vi "335 Read and Compressor auto control(SubVI).vi"(6 "压缩机自动停机":bool, 9 "自动控制":bool, 10 "数值":i32, 11 "Instrument":T1={"335 Resource"="", "Input (0:A)"=0, "Instrument Type"=enum."PPMS", "quantum design"=refnum, "Heater Output (1:1)"=0, "semaphore"=refnum, "TCP master instance"=refnum, "335 Status"=refnum, "M24C Resource"="GPIB0::24::INSTR", "4G supply"="GPIB0::24::INSTR", "Temp Status 24C"=refnum, "4g supply status"=refnum, "Temp"=refnum} {"Input (0:A)" items=["A", "B"]; "Heater Output (1:1)" items=["1"=1, "2"=2]}) -> (3 "簇":T5 {"?" items=["Unknow", "Stable", "Following Warm", "Following Cold", "Unfollowing"]})   [LabVIEW 2019, in "Get value.lvlib"]
uses:
  Get value.lvlib
  335 state.ctl
  Instrument.ctl
  <vilib>/NI/Modbus Library/API/Master/Modbus Master.lvclass
  Instrument Type.ctl
  lib/QDInstrument.dll
  lib/Lake Shore 335/Lake Shore 335.lvlib
panel:
  out "error out":errorcluster
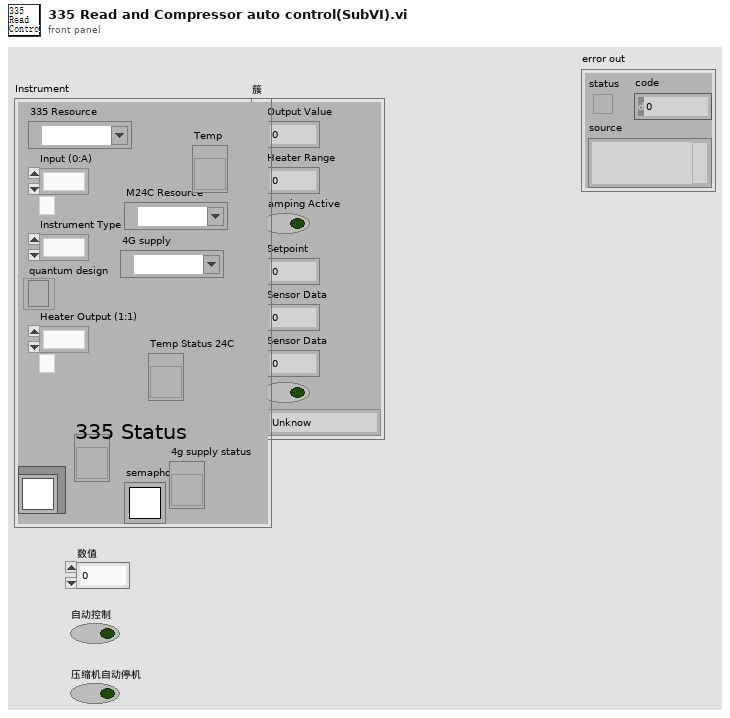
[diagram p1: front panel]
types:
  T1 = typedef "Instrument.ctl" = cluster{"335 Resource":refnum<visa-resource-name>, "Input (0:A)":u16, "Instrument Type":T2, "quantum design":refnum<k24>, "Heater Output (1:1)":u16, "semaphore":T3, "TCP master instance":refnum<class "Modbus Master.lvclass">, "335 Status":refnum<vi>, "M24C Resource":refnum<visa-resource-name>, "4G supply":refnum<visa-resource-name>, "Temp Status 24C":refnum<vi>, "4g supply status":refnum<vi>, "Temp":refnum<vi>}
  T2 = typedef "Instrument Type.ctl" = enum16{"PPMS", "VersaLab", "DynaCool", "SVSM", "PPMS-Rotate", "Lakeshore335", "9T mag"}
  T3 = typedef "Semaphore RefNum" = refnum<k1>
  T4 = typedef "335 state.ctl" = u16
  T5 = cluster{"Output Value":dbl, "Heater Range ":u16, "Ramping Active":bool, "Setpoint":dbl, "Sensor Data":dbl, "Sensor Data":dbl, bool, T4}
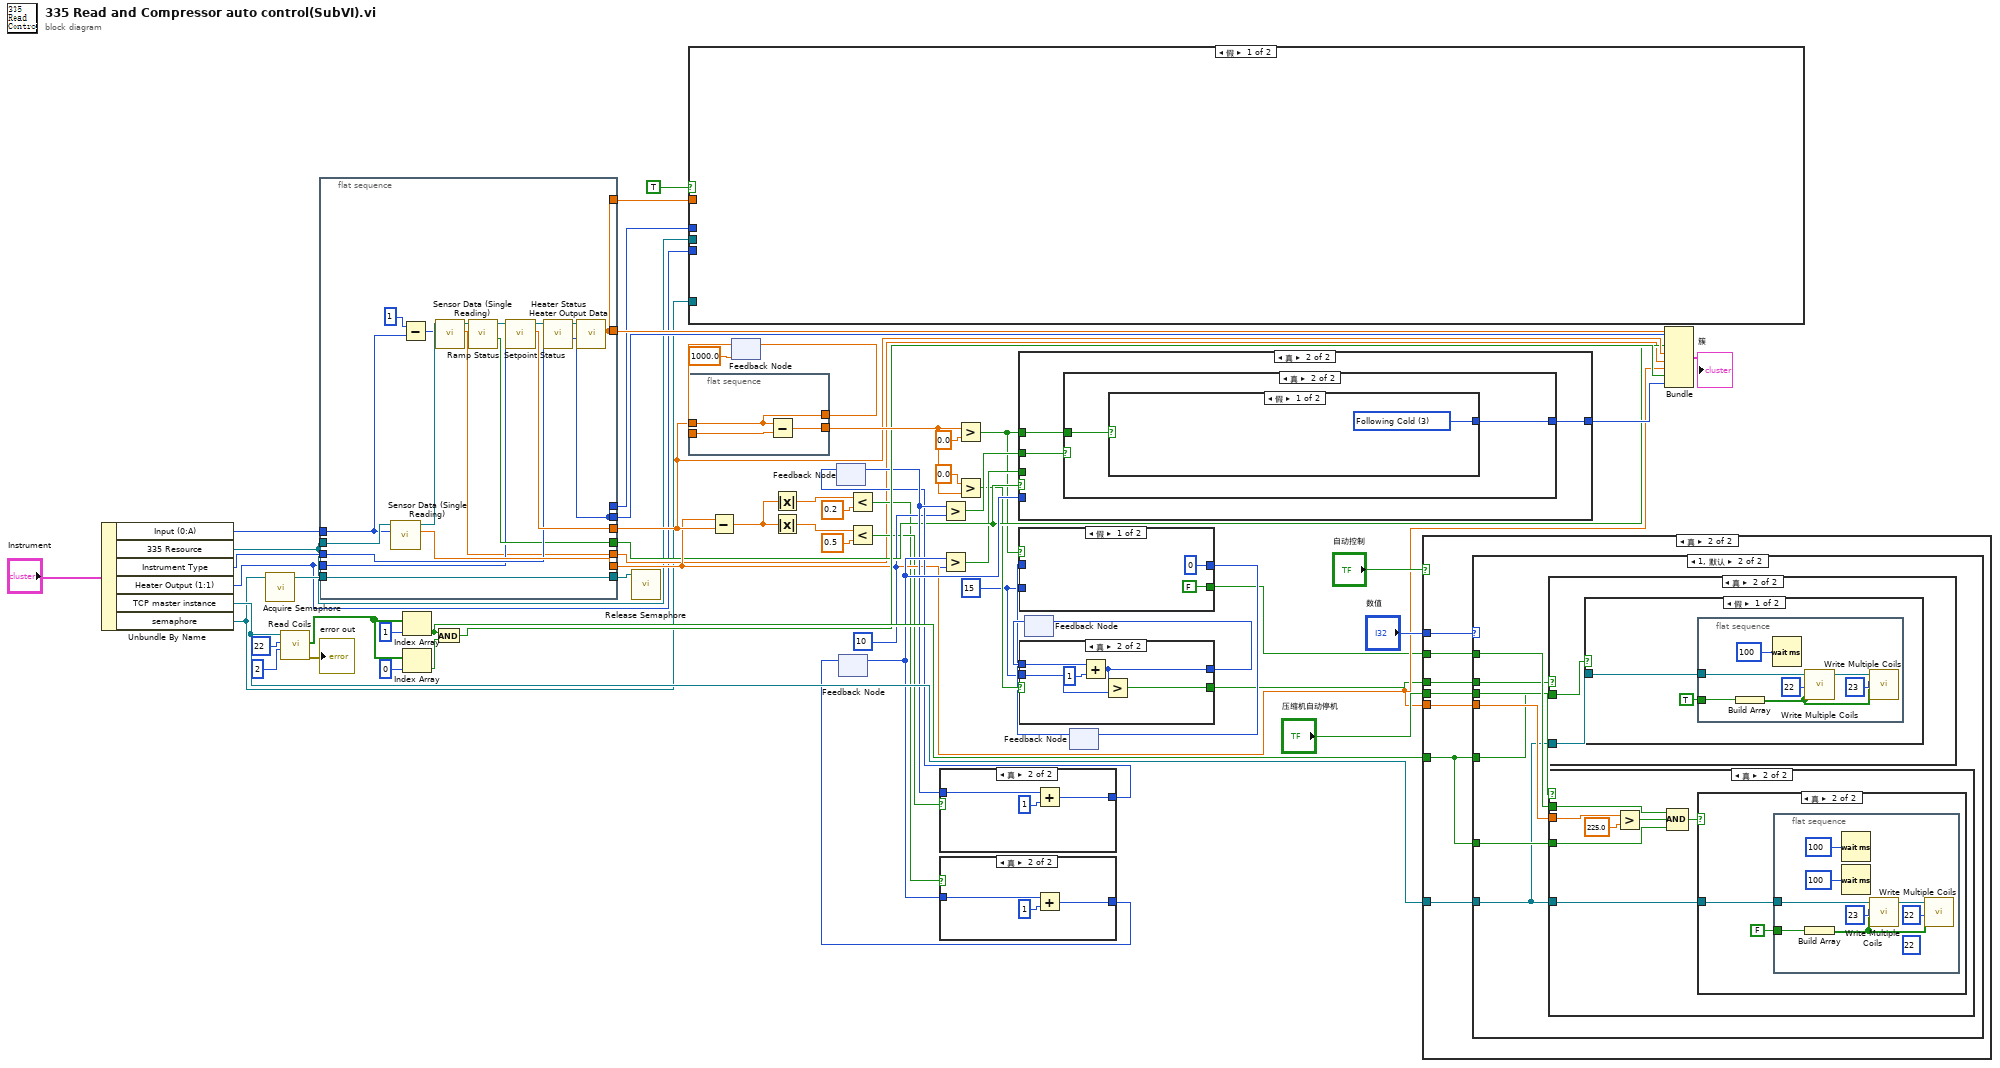
[diagram p0: block diagram]
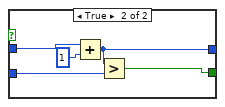
[diagram p2: hidden frame]
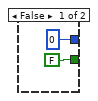
[diagram p3: hidden frame]
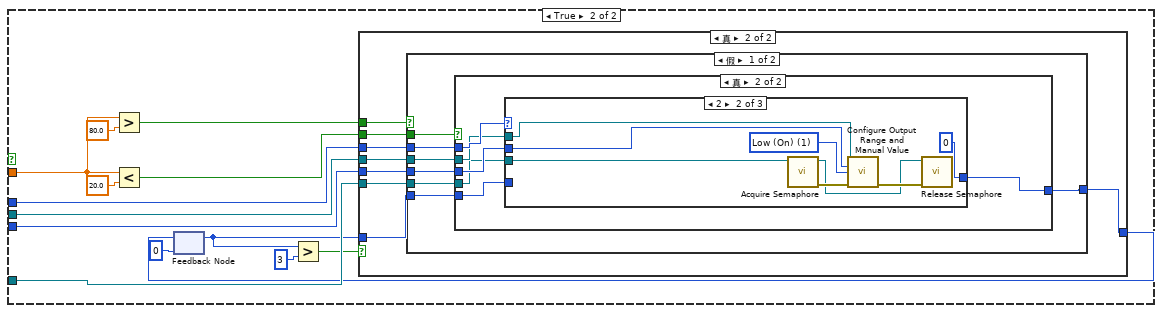
[diagram p4: hidden frame]
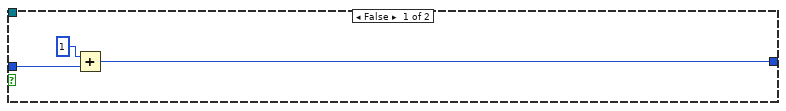
[diagram p5: hidden frame]
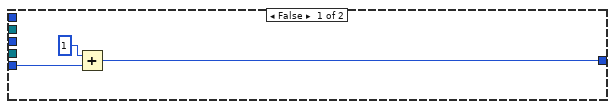
[diagram p6: hidden frame]
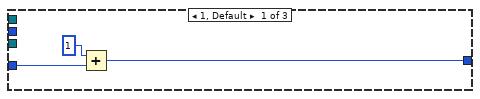
[diagram p7: hidden frame]
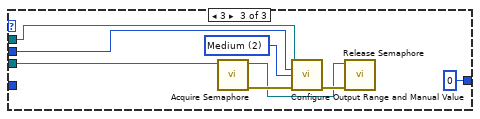
[diagram p8: hidden frame]
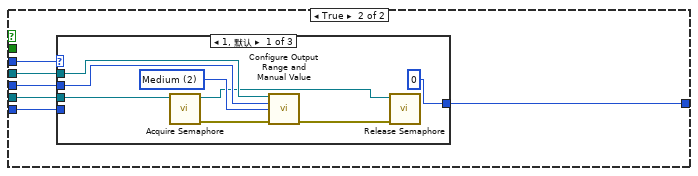
[diagram p9: hidden frame]
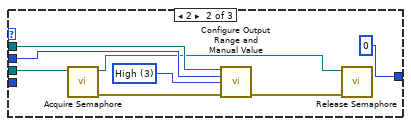
[diagram p10: hidden frame]
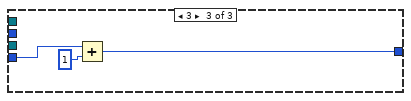
[diagram p11: hidden frame]
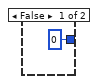
[diagram p18: hidden frame]
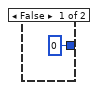
[diagram p19: hidden frame]
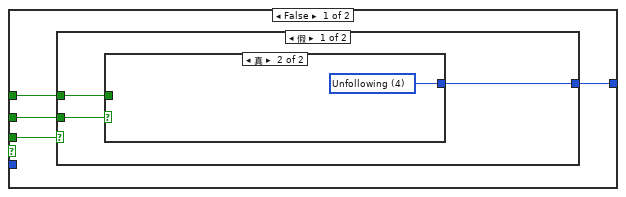
[diagram p20: hidden frame]
diagram:
  w2 = 15 ("y")
  w35 = 10 ("y")
  n1 = Unbundle By Name("Instrument") -> ("Input (0:A)"=w21:u16, "335 Resource"=w13:refnum<visa-resource-name>, "Instrument Type"=w18:T2, "Heater Output (1:1)"=w12:u16, "TCP master instance"=w59:refnum<class "Modbus Master.lvclass">, "semaphore"=w11:T3)
  n2 = call <vilib>:"Acquire Semaphore.vi"("semaphore"=w11) -> ("semaphore out"=w19:T3)  [unwired: 4 in, 2 out]
  n3 = call-dynamic "Read Coils.vi"("number of inputs"=u16 2, "starting address"=u16 22, "Modbus master in"=w59) -> ("error out"=→"error out":errorcluster, "coils"=w48:bool[])  [unwired: 6 in, 1 out]
  n4 = flat-sequence {
    tunnel: [w79] -> w49
    tunnel: w13 -> [w77]
    tunnel: [w74] -> w39
    tunnel: w18 -> [w73]
    tunnel: w19 -> [w72]
    tunnel: [w72] -> w20
    tunnel: [w62] -> w23
    tunnel: [w63] -> w22
    tunnel: [w71] -> w38
    tunnel: w12 -> [w70]
    tunnel: w21 -> [w69]
    tunnel: [w64] -> w24
    tunnel: [w63] -> w15
    tunnel: [w62] -> w14
    frame #0 {
      n5 = call "Sensor Data (Single Reading).vi"("Input (0:A)"=w69, "VISA resource name"=w77) -> ("Sensor Data"=w74:dbl, "VISA resource name out"=w67:refnum<visa-resource-name>)  [unwired: 7 in, 1 out]
      n6 = Subtract(x=u16 1, y=w69) -> (x-y=w65:u16)
      n7 = call "Sensor Data (Single Reading).vi"("Input (0:A)"=w65, "VISA resource name"=w67) -> ("Sensor Data"=w64:dbl, "VISA resource name out"=w66:refnum<visa-resource-name>)  [unwired: 7 in, 1 out]
      n8 = call "Ramp Status.vi"("VISA resource name"=w66) -> ("Ramping Active"=w71:bool, "VISA resource name out"=w78:refnum<visa-resource-name>)  [unwired: 6 in, 3 out]
      n9 = call "Setpoint Status.vi"("Output (1:1)"=w70, "VISA resource name"=w78) -> ("Setpoint"=w79:dbl, "VISA resource name out"=w76:refnum<visa-resource-name>)  [unwired: 7 in, 1 out]
      n10 = call "Heater Status.vi"("Heater Output (1:1)"=w73, "VISA resource name"=w76) -> ("Heater Range"=w62:u16, "VISA resource name out"=w75:refnum<visa-resource-name>)  [unwired: 5 in, 3 out]
      n11 = call "Heater Output Data.vi"("VISA resource name"=w75) -> ("Output Value"=w63:dbl)  [unwired: 8 in, 2 out]
    }
  }
  n12 = Index Array(array=w48, index=1) -> (element=w58:bool)
  n13 = Index Array(array=w48, index=0) -> (element=w44:bool)
  n14 = And(x=w58, y=w44) -> (x .and. y?=w45:bool)
  n15 = call <vilib>:"Release Semaphore.vi"("semaphore"=w20) -> ()  [unwired: 5 in, 2 out]
  n16 = case shown="假" TRUE {
    tunnel: w15 -> [_ w92]
    tunnel: w14 -> [_ w89]
    tunnel: w13 -> [_ w88]
    tunnel: w12 -> [_ w87]
    tunnel: w11 -> [_ w86]
    frame False {
    }
    frame True {
      n17 = Greater?(x=w92, y=80.0) -> (0:w90:bool)
      n18 = Less?(x=w92, y=20.0) -> (x < y?=w81:bool)
      n19 = feedback #1(0) -> (w82:i32)
      n20 = Greater?(x=w82, y=3) -> (0:w84:bool)
      n21 = case shown="真" w84 {
        tunnel: w90 -> [_ w104]
        tunnel: w89 -> [_ w103]
        tunnel: w88 -> [_ w102]
        tunnel: w87 -> [_ w101]
        tunnel: w86 -> [_ w100]
        tunnel: [w94 w99] -> w83
        tunnel: w82 -> [w96 w98]
        tunnel: w81 -> [_ w97]
        frame False {
          n22 = Add(x=1, y=w96) -> (x+y=w94:i32)
        }
        frame True {
          n23 = case shown="假" w104 {
            tunnel: w103 -> [w111 w145]
            tunnel: w102 -> [w110 w144]
            tunnel: w101 -> [w109 w143]
            tunnel: w100 -> [w106 w142]
            tunnel: [w108 w141] -> w99
            tunnel: w98 -> [w107 w140]
            tunnel: w97 -> [w105 _]
            frame False {
              n24 = case shown="真" w105 {
                tunnel: w111 -> [_ w120]
                tunnel: w110 -> [_ w119]
                tunnel: w109 -> [_ w118]
                tunnel: [w112 w117] -> w108
                tunnel: w107 -> [w114 w116]
                tunnel: w106 -> [_ w115]
                frame False {
                  n25 = Add(x=1, y=w114) -> (x+y=w112:i32)
                }
                frame True {
                  n26 = case shown="2" w120 {
                    tunnel: w119 -> [_ w127 w135]
                    tunnel: w118 -> [_ w126 w134]
                    tunnel: [w121 0 0] -> w117
                    tunnel: w116 -> [w123 _ _]
                    tunnel: w115 -> [_ w124 w132]
                    frame 1, Default {
                      n27 = Add(x=1, y=w123) -> (x+y=w121:i32)
                    }
                    frame 2 {
                      w131 = u16 1 items=["Off", "Low (On)", "Medium", "High"] ("Range (0:Off)")
                      n28 = call <vilib>:"Acquire Semaphore.vi"("semaphore"=w124) -> ("error out"=w130:errorcluster, "semaphore out"=w128:T3)  [unwired: 4 in, 1 out]
                      n29 = call "Configure Output Range and Manual Value.vi"("VISA resource name"=w127, "Heater Output (1:1)"=w126, "Range (0:Off)"=w131, "error in (no error)"=w130) -> ("error out"=w129:errorcluster)  [unwired: 10 in, 1 out]
                      n30 = call <vilib>:"Release Semaphore.vi"("error in (no error)"=w129, "semaphore"=w128) -> ()  [unwired: 4 in, 2 out]
                    }
                    frame 3 {
                      w139 = u16 2 items=["Off", "Low (On)", "Medium", "High"] ("Range (0:Off)")
                      n31 = call <vilib>:"Acquire Semaphore.vi"("semaphore"=w132) -> ("error out"=w138:errorcluster, "semaphore out"=w136:T3)  [unwired: 4 in, 1 out]
                      n32 = call "Configure Output Range and Manual Value.vi"("VISA resource name"=w135, "Heater Output (1:1)"=w134, "Range (0:Off)"=w139, "error in (no error)"=w138) -> ("error out"=w137:errorcluster)  [unwired: 10 in, 1 out]
                      n33 = call <vilib>:"Release Semaphore.vi"("error in (no error)"=w137, "semaphore"=w136) -> ()  [unwired: 4 in, 2 out]
                    }
                  }
                }
              }
            }
            frame True {
              n34 = case shown="1, 默认" w145 {
                tunnel: w144 -> [w153 w161 _]
                tunnel: w143 -> [w152 w160 _]
                tunnel: w142 -> [w146 w155 _]
                tunnel: [0 0 w162] -> w141
                tunnel: w140 -> [_ _ w164]
                frame 1, Default {
                  w149 = u16 2 items=["Off", "Low (On)", "Medium", "High"] ("Range (0:Off)")
                  n35 = call <vilib>:"Acquire Semaphore.vi"("semaphore"=w146) -> ("error out"=w150:errorcluster, "semaphore out"=w148:T3)  [unwired: 4 in, 1 out]
                  n36 = call "Configure Output Range and Manual Value.vi"("VISA resource name"=w153, "Heater Output (1:1)"=w152, "Range (0:Off)"=w149, "error in (no error)"=w150) -> ("error out"=w151:errorcluster)  [unwired: 10 in, 1 out]
                  n37 = call <vilib>:"Release Semaphore.vi"("error in (no error)"=w151, "semaphore"=w148) -> ()  [unwired: 4 in, 2 out]
                }
                frame 2 {
                  w159 = u16 3 items=["Off", "Low (On)", "Medium", "High"] ("Range (0:Off)")
                  n38 = call <vilib>:"Acquire Semaphore.vi"("semaphore"=w155) -> ("error out"=w158:errorcluster, "semaphore out"=w156:T3)  [unwired: 4 in, 1 out]
                  n39 = call "Configure Output Range and Manual Value.vi"("VISA resource name"=w161, "Heater Output (1:1)"=w160, "Range (0:Off)"=w159, "error in (no error)"=w158) -> ("error out"=w157:errorcluster)  [unwired: 10 in, 1 out]
                  n40 = call <vilib>:"Release Semaphore.vi"("error in (no error)"=w157, "semaphore"=w156) -> ()  [unwired: 4 in, 2 out]
                }
                frame 3 {
                  n41 = Add(x=w164, y=1) -> (x+y=w162:i32)
                }
              }
            }
          }
        }
      }
      n42 = feedback-in #1(w83) -> ()
    }
  }
  n43 = flat-sequence {
    tunnel: w49 -> [w167]
    tunnel: [w167] -> w50
    tunnel: w51 -> [w166]
    tunnel: [w165] -> w57
    frame #0 {
      n44 = Subtract(x=w167, y=w166) -> (x-y=w165:dbl)
    }
  }
  n45 = Subtract(x=w39, y=w49) -> (x-y=w33:dbl)
  n46 = feedback #2(1000.0 ("Setpoint")) -> (w51:dbl)
  n47 = feedback-in #2(w50) -> ()
  n48 = Absolute Value(x=w33) -> (abs(x)=w30:dbl)
  n49 = Absolute Value(x=w33) -> (abs(x)=w31:dbl)
  n50 = feedback #3() -> (w41:i32)  [unwired: 1 in]
  n51 = feedback #4() -> (w43:i32)  [unwired: 1 in]
  n52 = Less?(x=w30, y=0.2) -> (x < y?=w29:bool)
  n53 = Less?(x=w31, y=0.5) -> (x < y?=w34:bool)
  n54 = case shown="真" w34 {
    tunnel: w41 -> [_ w171]
    tunnel: [0 w169] -> w40
    frame False {
    }
    frame True {
      n55 = Add(x=w171, y=1) -> (x+y=w169:i32)
    }
  }
  n56 = feedback-in #3(w40) -> ()
  n57 = case shown="真" w29 {
    tunnel: w43 -> [_ w175]
    tunnel: [0 w173] -> w42
    frame False {
    }
    frame True {
      n58 = Add(x=w175, y=1) -> (x+y=w173:i32)
    }
  }
  n59 = feedback-in #4(w42) -> ()
  n60 = Greater?(x=w41, y=w35) -> (0:w37:bool)
  n61 = Greater?(x=w43, y=w35) -> (0:w36:bool)
  n62 = Greater?(x=w57, y=0.0) -> (0:w4:bool)
  n63 = Greater?(x=0.0, y=w57) -> (0:w9:bool)
  n64 = case shown="真" w38 {
    tunnel: w43 -> [_ _]
    tunnel: w36 -> [w179 _]
    tunnel: w37 -> [w178 w188]
    tunnel: [w177 w187] -> w54
    tunnel: w4 -> [w176 w186]
    frame False {
      n65 = case shown="假" w179 {
        tunnel: [w181 w185] -> w177
        tunnel: w178 -> [w182 _]
        tunnel: w176 -> [w180 _]
        frame False {
          n66 = case shown="真" w182 {
            tunnel: [w183 w184] -> w181
            tunnel: w180 -> [_ _]
            frame False {
              w183 = T4 4 items=["Unknow", "Stable", "Following Warm", "Following Cold", "Unfollowing"]
            }
            frame True {
              w184 = T4 4 items=["Unknow", "Stable", "Following Warm", "Following Cold", "Unfollowing"]
            }
          }
        }
        frame True {
          w185 = T4 1 items=["Unknow", "Stable", "Following Warm", "Following Cold", "Unfollowing"]
        }
      }
    }
    frame True {
      n67 = case shown="真" w188 {
        tunnel: [w189 w190] -> w187
        tunnel: w186 -> [_ w191]
        frame False {
          w189 = T4 4 items=["Unknow", "Stable", "Following Warm", "Following Cold", "Unfollowing"]
        }
        frame True {
          n68 = case shown="假" w191 {
            tunnel: [w192 w193] -> w190
            frame False {
              w192 = T4 3 items=["Unknow", "Stable", "Following Warm", "Following Cold", "Unfollowing"]
            }
            frame True {
              w193 = T4 2 items=["Unknow", "Stable", "Following Warm", "Following Cold", "Unfollowing"]
            }
          }
        }
      }
    }
  }
  n69 = feedback #5() -> (w7:i32)  [unwired: 1 in]
  n70 = case shown="真" w9 {
    tunnel: [0 w198] -> w8
    tunnel: w7 -> [_ w199]
    tunnel: w2 -> [_ w197]
    tunnel: [FALSE w196] -> w3
    frame False {
    }
    frame True {
      n71 = Add(x=w199, y=1) -> (x+y=w198:i32)
      n72 = Greater?(x=w198, y=w197) -> (0:w196:bool)
    }
  }
  n73 = feedback-in #5(w8) -> ()
  n74 = feedback #6() -> (w6:i32)  [unwired: 1 in]
  n75 = case shown="假" w4 {
    tunnel: [0 w204] -> w5
    tunnel: w6 -> [_ w206]
    tunnel: w2 -> [_ w205]
    tunnel: [FALSE w203] -> w1
    frame False {
    }
    frame True {
      n76 = Add(x=w206, y=1) -> (x+y=w204:i32)
      n77 = Greater?(x=w204, y=w205) -> (0:w203:bool)
    }
  }
  n78 = feedback-in #6(w5) -> ()
  n79 = case shown="真" "自动控制" {
    tunnel: w39 -> [_ w214]
    tunnel: w1 -> [_ w213]
    tunnel: "压缩机自动停机" -> [_ w212]
    tunnel: "数值" -> [_ w211]
    tunnel: w3 -> [_ w210]
    tunnel: w58 -> [_ w209]
    tunnel: w59 -> [_ w208]
    frame False {
    }
    frame True {
      n80 = case shown="1, 默认" w211 {
        tunnel: w214 -> [_ w221]
        tunnel: w213 -> [_ w220]
        tunnel: w209 -> [_ w219]
        tunnel: w212 -> [_ w218]
        tunnel: w210 -> [_ w217]
        tunnel: w209 -> [_ w216]
        tunnel: w208 -> [_ w215]
        frame 0 {
        }
        frame 1, Default {
          n81 = case shown="真" w217 {
            tunnel: w216 -> [_ w223]
            tunnel: w215 -> [_ w222]
            frame False {
            }
            frame True {
              n82 = case shown="假" w223 {
                tunnel: w222 -> [w224 _]
                frame False {
                  n83 = flat-sequence {
                    tunnel: TRUE -> [w228]
                    tunnel: w224 -> [w231]
                    frame #0 {
                      n84 = Build Array(w228) -> (w227:bool[])
                      n85 = Wait (ms)(milliseconds to wait=u32 100 ("等待时间（毫秒）")) -> ()  [unwired: 1 out]
                      n86 = call-dynamic "Write Multiple Coils.vi"("coils to write"=w227, "starting address"=u16 22, "Modbus master in"=w231) -> ("Modbus master out"=w229:refnum<class "Modbus Master.lvclass">)  [unwired: 7 in, 1 out]
                      n87 = call-dynamic "Write Multiple Coils.vi"("coils to write"=w227, "starting address"=u16 23, "Modbus master in"=w229) -> ()  [unwired: 7 in, 2 out]
                    }
                  }
                }
                frame True {
                }
              }
            }
          }
          n88 = case shown="真" w218 {
            tunnel: w221 -> [_ w239]
            tunnel: w220 -> [_ w237]
            tunnel: w219 -> [_ w236]
            tunnel: w215 -> [_ w233]
            frame False {
            }
            frame True {
              n89 = Greater?(x=w239, y=225.0) -> (0:w235:bool)
              n90 = Compound Arithmetic op=AND ("复合运算")(w237, w235, w236) -> (w234:bool)
              n91 = case shown="真" w234 {
                tunnel: w233 -> [_ w240]
                frame False {
                }
                frame True {
                  n92 = flat-sequence {
                    tunnel: FALSE -> [w245]
                    tunnel: w240 -> [w244]
                    frame #0 {
                      (unwired) u16 22 ("starting address")
                      n93 = Build Array(w245) -> (w242:bool[])
                      n94 = Wait (ms)(milliseconds to wait=u32 100 ("等待时间（毫秒）")) -> ()  [unwired: 1 out]
                      n95 = Wait (ms)(milliseconds to wait=u32 100 ("等待时间（毫秒）")) -> ()  [unwired: 1 out]
                      n96 = call-dynamic "Write Multiple Coils.vi"("coils to write"=w242, "starting address"=u16 23, "Modbus master in"=w244) -> ("Modbus master out"=w243:refnum<class "Modbus Master.lvclass">)  [unwired: 7 in, 1 out]
                      n97 = call-dynamic "Write Multiple Coils.vi"("coils to write"=w242, "starting address"=u16 22, "Modbus master in"=w243) -> ()  [unwired: 7 in, 2 out]
                    }
                  }
                }
              }
            }
          }
        }
      }
    }
  }
  n98 = Bundle("Output Value"=w22, "Heater Range"=w23, "Ramping Active"=w38, "Setpoint"=w49, "Sensor Data"=w24, "Sensor Data"=w39, w45, w54) -> (→"簇":T5)  [unwired: 1 in]
